vi "mcc_etc_DIO_open.vi"(10 "input_line":refnum<k21>="Dev2/AuxPort/Di4", 11 "output_line":refnum<k21>) -> (0 "error out":errorcluster, 1 "status":bool=TRUE, 2 "input_task_out":refnum<k24>, 3 "output_task out":refnum<k24>)   [LabVIEW 2019]
uses:
  C:/Program Files/National Instruments/LabVIEW 2019/vi.lib/ULx/ULx_LV.dll
  Program Files/National Instruments/LabVIEW 2019/vi.lib/ULx/ULx_LV.dll
  <vilib>/ULx/Create Channel.llb/ULx Create Channel (DO-Digital Output).vi
  <vilib>/ULx/Create Channel.llb/ULx Create Channel (DI-Digital Input).vi
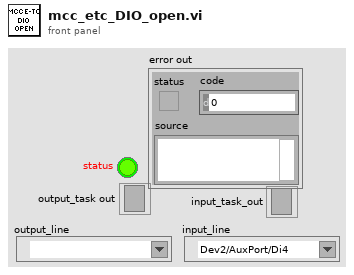
[diagram p1: front panel]
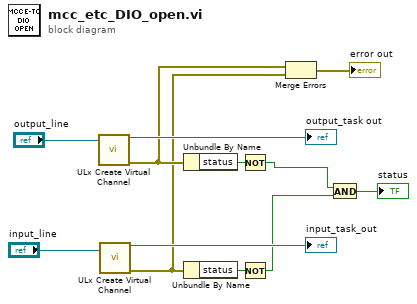
[diagram p0: block diagram]
diagram:
  n1 = call-poly <vilib>:"ULx Create Virtual Channel.vi"("lines"="output_line") -> ("task out"=→"output_task out":refnum<k24>, "error out"=w3:errorcluster)  [unwired: 13 in]
  n2 = call-poly <vilib>:"ULx Create Virtual Channel.vi"("lines"="input_line") -> ("task out"=→"input_task_out":refnum<k24>, "error out"=w2:errorcluster)  [unwired: 13 in]
  n3 = Unbundle By Name(w3) -> ("status"=w11:bool)
  n4 = Unbundle By Name(w2) -> ("status"=w7:bool)
  n5 = Not(x=w11) -> (.not. x?=w5:bool)
  n6 = Not(x=w7) -> (.not. x?=w6:bool)
  n7 = Merge Errors(w3, w2) -> (→"error out":errorcluster)
  n8 = And(x=w5, y=w6) -> (x .and. y?=→"status":bool)
